vi "Initialize.vi"(0 "instance":u8) -> (4 "subsysytem":refnum<class "Single Address Space Collection.lvclass">, 6 "AddressSpace":refnum<class "AddressSpace.lvclass">)   [LabVIEW 2017, in "ActiveFrontEnd.lvlib" / "AddressSpace.lvclass"]
uses:
  AddressSpace.lvclass
  C:/Program Files (x86)/National Instruments/LabVIEW 2017/instr.lib/_niInstr/Instruction Framework/v1/FPGA/Interfaces/Address Space/Address Space.lvclass
  <instrlib>/_niInstr/Instruction Framework/v1/FPGA/Helper Classes/Single Address Space Collection/Single Address Space Collection.lvclass
  AddressSpace.lvclass/AddressSpace.ctl
  <vilib>/rvi/eio/common/nirviEmuReportErrorAndStop.vi
  <vilib>/rvi/DataTransferAndStorage/Container/Common/niFpgaContainerSetEmuInfo.vi
  <vilib>/rvi/DataTransferAndStorage/Container/Common/niFpgaContainerGetUniqueNameForEmu.vi
  <vilib>/rvi/LocalResourceManager/LocalResourceManager.xnode
  ActiveFrontEnd.lvlib
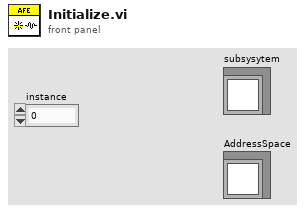
[diagram p1: front panel]
types:
  T1 = typedef "ActiveFrontEnd.lvlib/ControllerRegisters.ctl" = cluster{"Range":refnum<k21>, "Gains":refnum<k21>, "Setpoints":refnum<k21>, "Signals":refnum<k21>, "Parameters":refnum<k21>, "ManualControl":refnum<k21>}
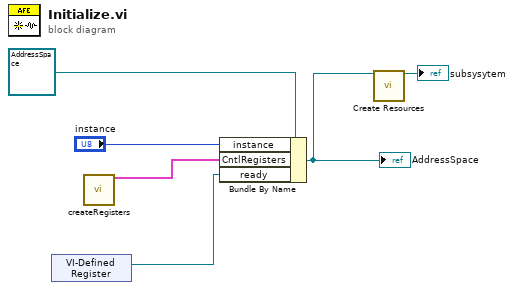
[diagram p0: block diagram]
diagram:
  n1 = xnode "VI-Defined Register"() -> ("Register Out"=w1:refnum<k21>)
  n2 = call "createRegisters.vi"() -> ("ControllerRegisters"=w4:T1)  [unwired: 15 in]
  n3 = Bundle By Name(cluster=refnum<class "AddressSpace.lvclass"> refnum ("ActiveFrontEnd.lvlib:AddressSpace.lvclass"), "instance"="instance", "CntlRegisters"=w4, "ready"=w1) -> (w3:refnum<class "AddressSpace.lvclass">)
  "AddressSpace" <- w3
  n4 = call <instrlib>:"Create Resources.vi"("address space"=w3) -> ("single address space collection"=→"subsysytem":refnum<class "Single Address Space Collection.lvclass">)  [unwired: 14 in]
